vi "DIMPowerSupply.contents.vi"() -> ()   [LabVIEW 2014, in "DIMPowerSupply.lvlib"]
doc: "loads all VIs into memory - required for building an application"
uses:
  DIMPowerSupply.lvlib
panel:
  out "error out":errorcluster
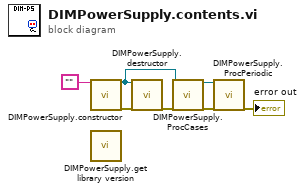
[diagram p0: block diagram]
diagram:
  n1 = call "DIMPowerSupply.constructor.vi"("name"="") -> ("i ref out"=w5:refnum<vi>, "error out"=w4:errorcluster)  [unwired: 16 in, 1 out]
  n2 = call "DIMPowerSupply.get library version.vi"() -> ()  [unwired: 1 in, 1 out]
  n3 = call "DIMPowerSupply.destructor.vi"("i ref in"=w5, "error in (no error)"=w4) -> ("error out"=w3:errorcluster)  [unwired: 17 in]
  n4 = call "DIMPowerSupply.ProcCases.vi"("i ref in"=w5, "error in (no error)"=w3) -> ("i ref out"=w7:refnum<vi>, "error out"=w2:errorcluster)  [unwired: 15 in, 1 out]
  n5 = call "DIMPowerSupply.ProcPeriodic.vi"("i ref in"=w7, "error in (no error)"=w2) -> ("error out"=→"error out":errorcluster)  [unwired: 15 in, 2 out]
